vi "HIOKI PW3390 Conf CH A.vi"   [LabVIEW 2009]
doc: "Sets and reads the functions related to the Motor Analysis Option's Channel A. CH A input can select either AnalogDC or Frequency."
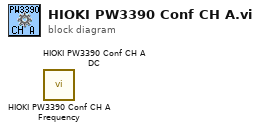
[diagram p0: block diagram]
diagram:
  n1 = call <instrlib>:"HIOKI PW3390 Conf CH A Frequency.vi"() -> ()  [unwired: 10 in, 6 out]
  n2 = call <instrlib>:"HIOKI PW3390 Conf CH A DC.vi"() -> ()  [unwired: 10 in, 6 out]
